vi "U16 Array to Double.vi"(10 "U16 Array":u16[](array[numeric])) -> (2 "Double":dbl)   [LabVIEW 2015, in "Modbus Data Conversion.lvlib"]
uses:
  Modbus Data Conversion.lvlib
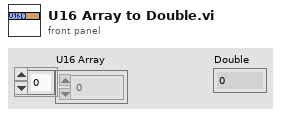
[diagram p1: front panel]
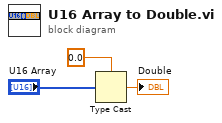
[diagram p0: block diagram]
diagram:
  n1 = Type Cast(type=0.0 ("Double"), x="U16 Array") -> (*(type *) &x=→"Double":dbl)
